vi "Set Descriptions.vi"(0 "Robot Arm in":refnum<class "Robot Arm.lvclass">, 5 "Name":string, 7 "Manufacturer":string, 9 "Comment":string, 11 "error in (no error)":errorcluster) -> (4 "Robot Arm out":refnum<class "Robot Arm.lvclass">, 15 "error out":errorcluster)   [LabVIEW 2013, in "Robot Arm.lvclass"]
uses:
  Robot Arm.lvclass
  Robot Arm.lvclass/Robot Arm.ctl
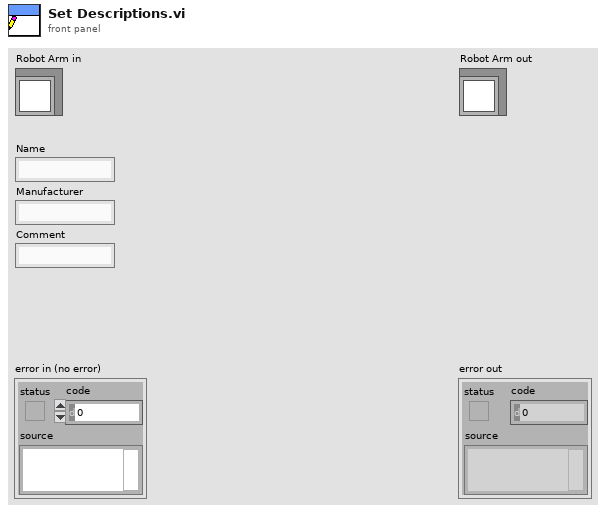
[diagram p1: front panel]
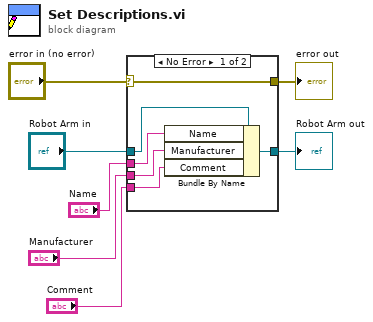
[diagram p0: block diagram]
diagram:
  n1 = case shown="No Error" "error in (no error)" {
    selector: "error in (no error)" -> [w13 w14]
    tunnel: [w13 w14] -> w6
    tunnel: [w11 w15] -> w4
    tunnel: "Robot Arm in" -> [w12 w15]
    tunnel: "Name" -> [w10 _]
    tunnel: "Manufacturer" -> [w9 _]
    tunnel: "Comment" -> [w8 _]
    frame No Error {
      n2 = Bundle By Name(cluster=w12, "Name"=w10, "Manufacturer"=w9, "Comment"=w8) -> (w11:refnum<class "Robot Arm.lvclass">)
    }
    frame Error {
    }
  }
  "error out" <- w6
  "Robot Arm out" <- w4
